vi "configuration UI.vi"() -> ()   [LabVIEW 2013, in "tag bus configurable plugin editor node.lvclass"]
uses:
  tag bus configurable plugin editor node.lvclass
  <vilib>/CEF_TreeControl/Node/NodeRef.ctl
  <vilib>/CEF_TreeControl/Node/NISE_CEF_Node.lvclass
  <vilib>/NI/AMC/Message Queue.ctl
  <vilib>/NI/AMC/Message.ctl
  <vilib>/NI/Tools/Keyed Array/KeyedArray.ctl
  <vilib>/CEF_TreeControl/Node/UserEventRef.ctl
  <vilib>/CEF_TreeControl/Controls/EventCluster.ctl
  module/configuration/tag bus configurable plugin module configuration.lvclass
  <vilib>/NI/Tag Bus Data Framework/Configuration Editor/Classes/Engine Parent/Engine Parent Editor Node.lvclass
  <vilib>/NI/Tag Bus/tag/tag descriptor.lvclass
  <vilib>/NI/Tag Bus/tag/Data Type.ctl
  <vilib>/NI/Module Execution Interface/Engine Configuration/engine configuration.lvclass
  <vilib>/NI/Tag Bus/tag/tag descriptor.lvclass/tag descriptor.ctl
  tag bus configurable plugin editor node.lvclass/tag bus configurable plugin editor node.ctl
  <vilib>/NI/Tag Bus Module Framework/root configuration/TBM configuration.lvclass/TBM configuration.ctl
  <vilib>/NI/Tag Bus/tag/write tag name.vi
  <vilib>/NI/Tag Bus/tag/write data type.vi
  <vilib>/NI/Tag Bus Module Framework/root configuration/create GUID.vi
  <vilib>/CEF_TreeControl/NISE_CEF_TreeControl.lvlib
  <vilib>/NI/Tag Bus Data Framework/Configuration Editor/Classes/Module editor node/module editor node.lvclass
  <vilib>/NI/Tag Bus Module Framework/channel/TBM channel.lvclass
  <vilib>/NI/Tag Bus Module Framework/root configuration/TBM configuration.lvclass
  <vilib>/NI/Tools/Keyed Array/Tools_KeyedArray.lvlib
  <vilib>/NI/AMC/AMC.lvlib
panel:
  in  "Tab Control":enum32{"Static Configuration"}(tab)
  in  "hidden_remove":bool
  in  "hidden_settings":bool
  in  "hidden_Add":bool
  in  "Remove Button":bool
  in  "Add Button":bool
  in  "channel":i32(listbox)
  in  "settings":bool
  in  "user event":T1
  in  "main queue":T2
  in  "node ref":T3
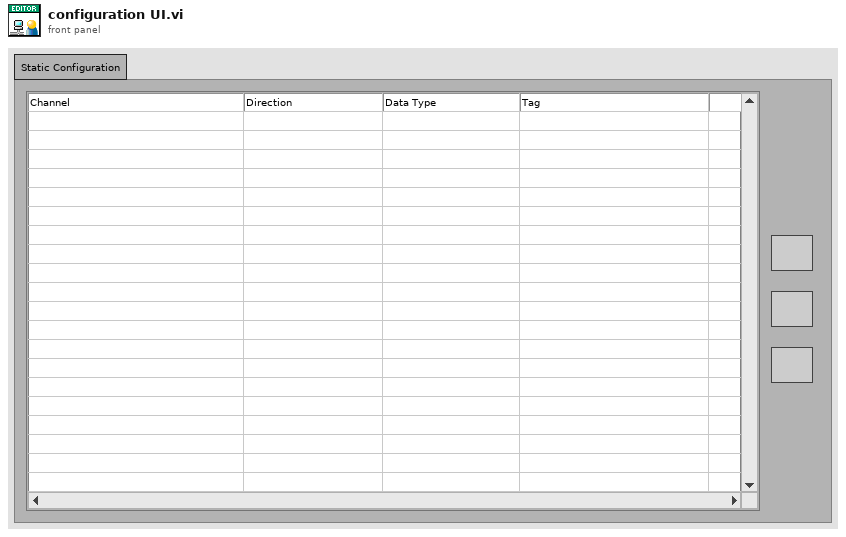
[diagram p1: front panel]
types:
  T1 = typedef "NISE_CEF_Node.lvclass/UserEventRef.ctl" = refnum<user-event>
  T2 = typedef "AMC.lvlib/Message Queue.ctl" = refnum<queue>
  T3 = typedef "NISE_CEF_Node.lvclass/NodeRef.ctl" = refnum<data-value>
  T4 = typedef "NISE_CEF_TreeControl.lvlib/EventCluster.ctl" = cluster{"command":string, "data":string}
  T5 = typedef "tag bus.lvlib/tag descriptor.lvclass/Data Type.ctl" = enum16{"Double", "Single", "I64", "I32", "I16", "I8", "U64", "U32", "U16", "U8", "Boolean", "String", "Array of Double", "Array of Single", "Array of I64", "Array of I32", "Array of I16", "Array of I8", "Array of U64", "Array of U32", "Array of U16", "Array of U8", "Array of Boolean", "Array of String"}
  T6 = typedef "tag bus configurable plugin editor node.lvclass/table line.ctl" = cluster{"channel":refnum<class "TBM channel.lvclass">, "tag name":string}
  T7 = typedef "LVPoint32TypeDef.ctl" = cluster{"Horizontal":i32, "Vertical":i32}
  T8 = typedef "LVRowAndColumnTypeDef.ctl" = cluster{"Row":i32, "Column":i32}
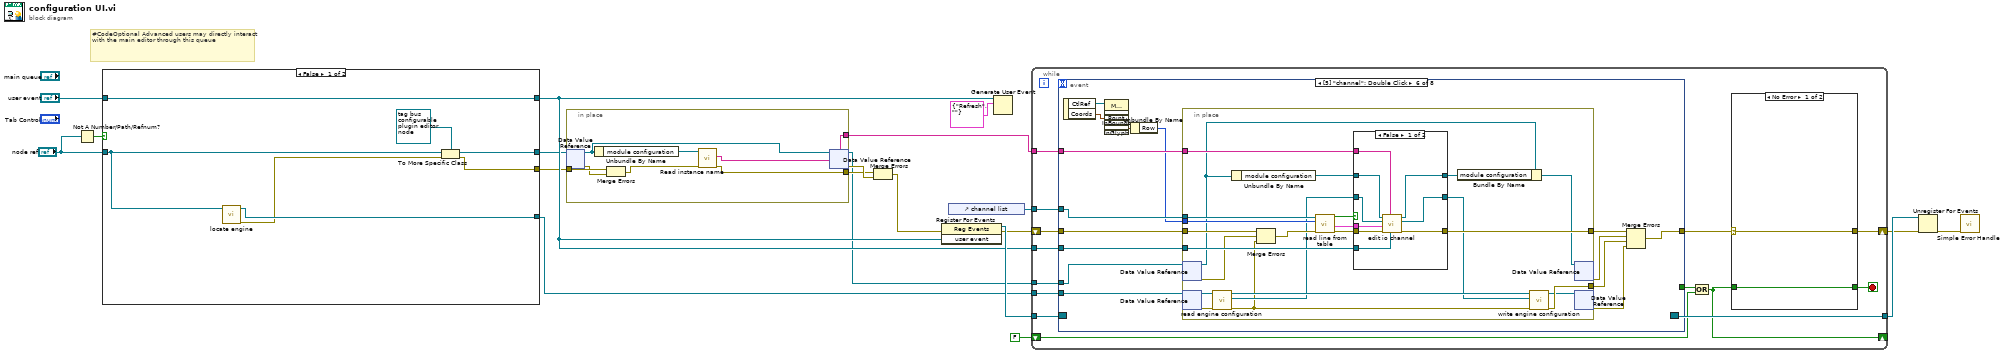
[diagram p0: block diagram]
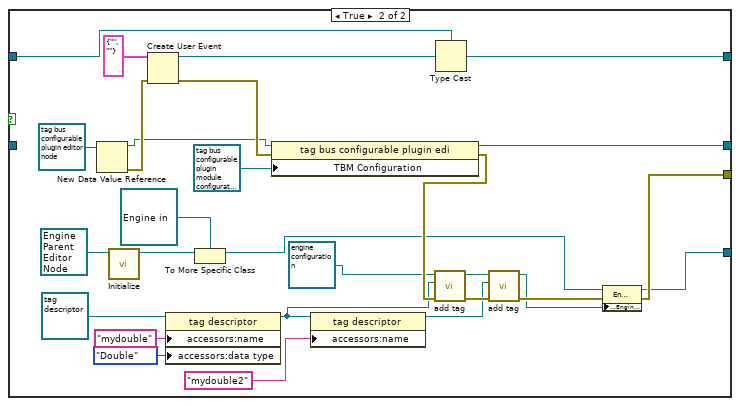
[diagram p2: hidden frame]
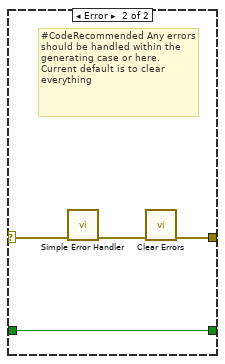
[diagram p3: hidden frame]
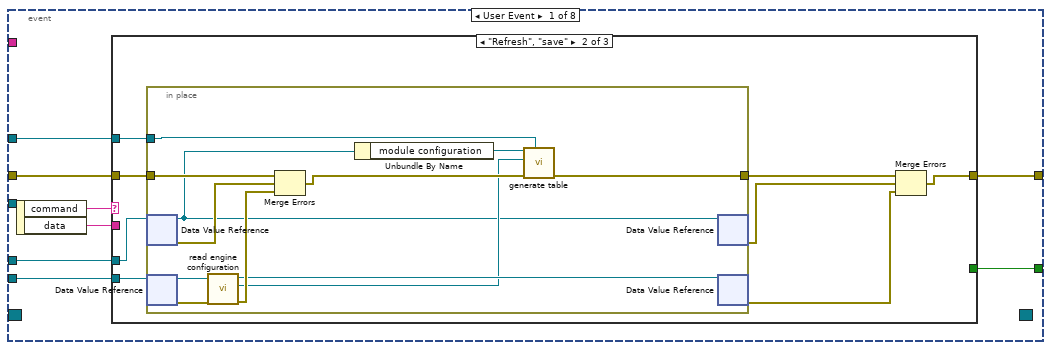
[diagram p4: hidden frame]
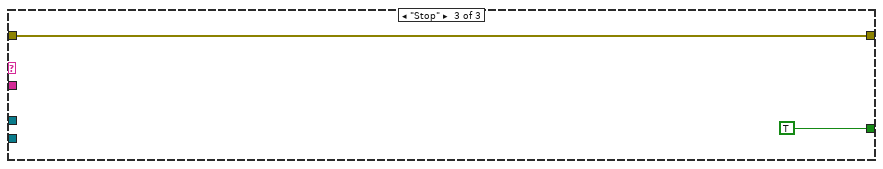
[diagram p6: hidden frame]
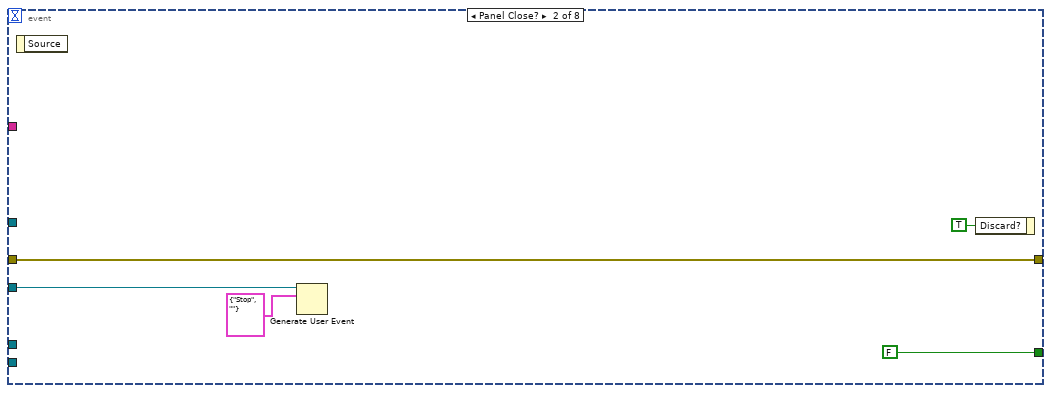
[diagram p7: hidden frame]
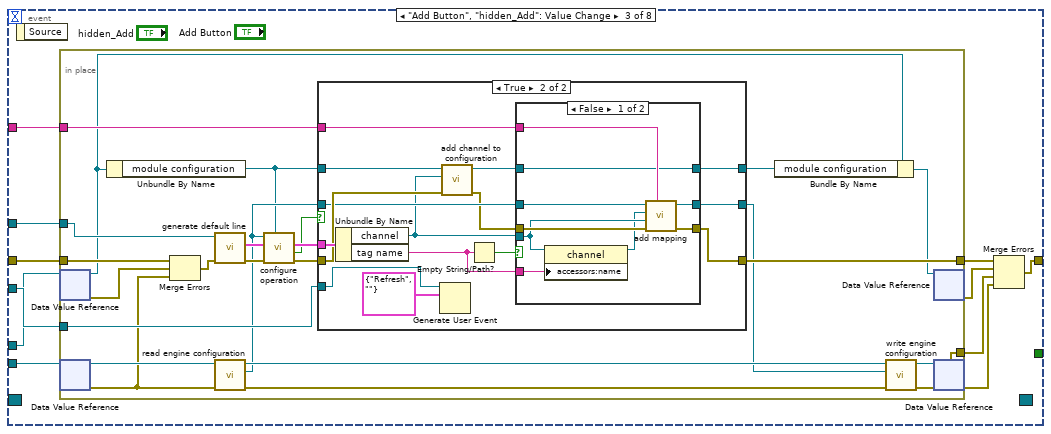
[diagram p8: hidden frame]
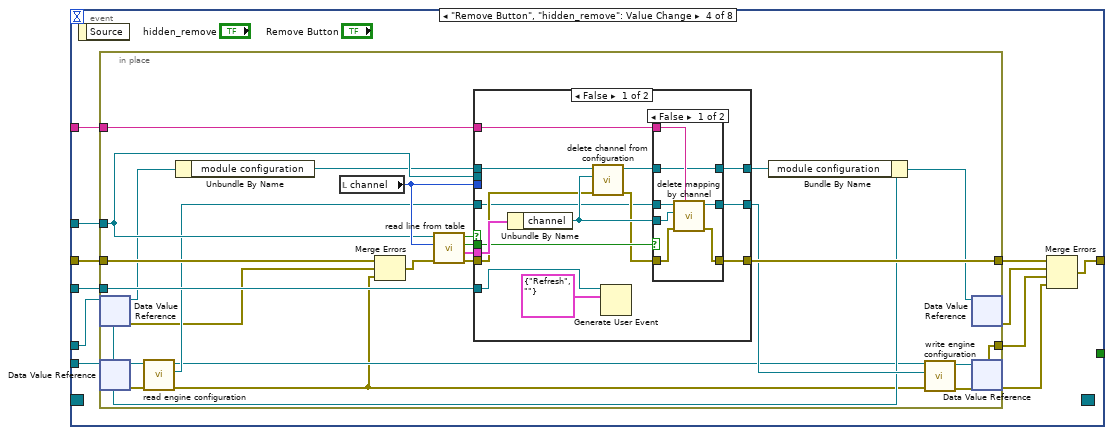
[diagram p11: hidden frame]
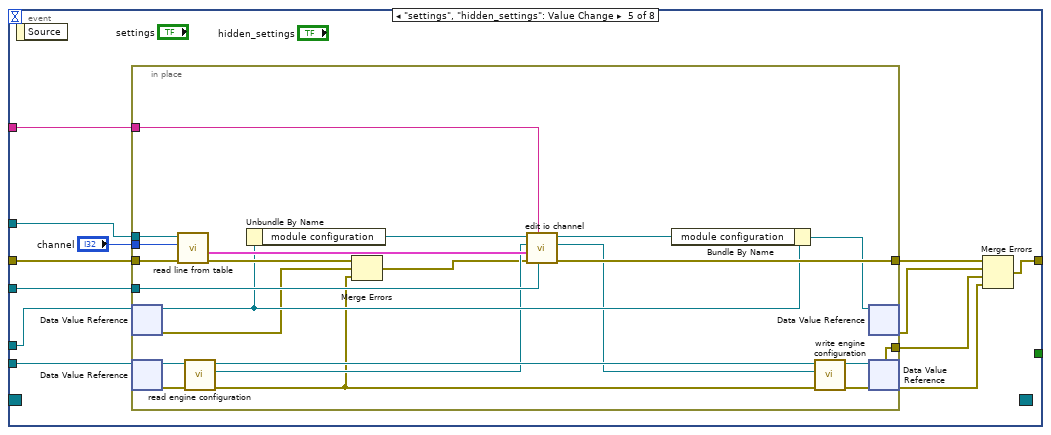
[diagram p14: hidden frame]
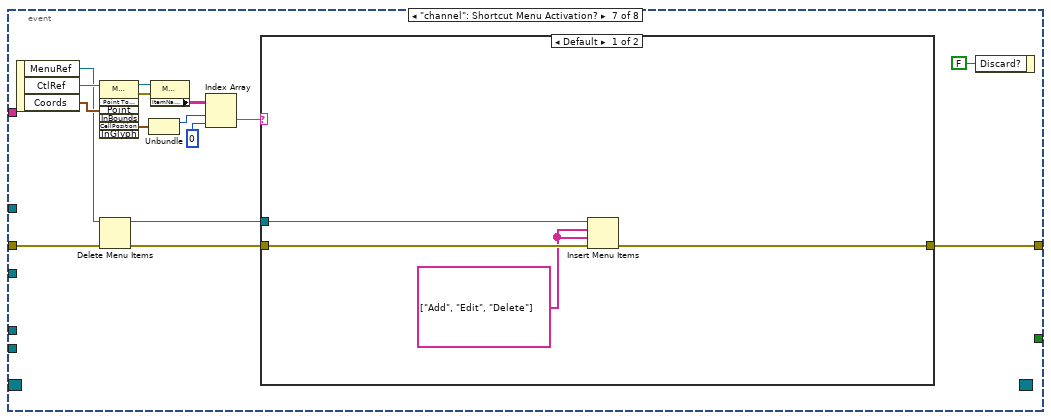
[diagram p16: hidden frame]
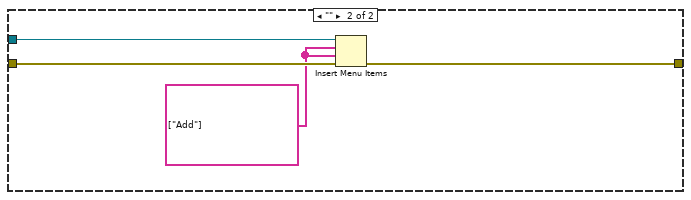
[diagram p17: hidden frame]
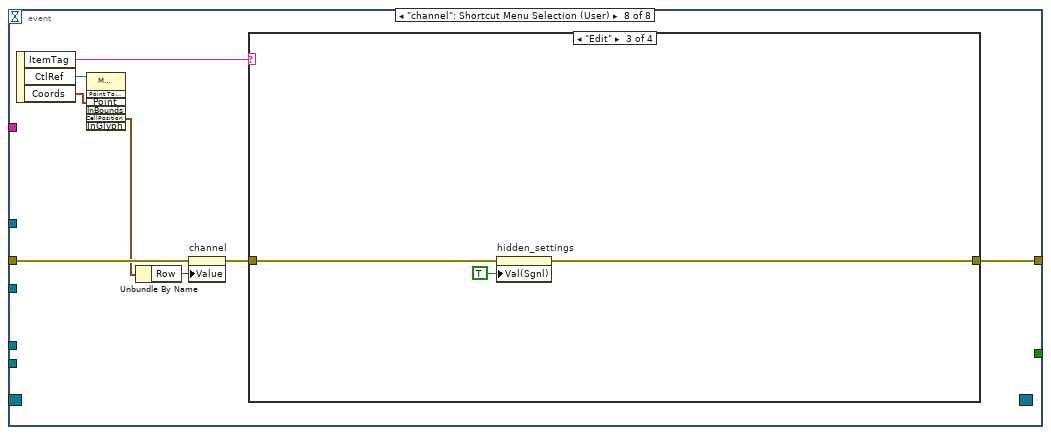
[diagram p18: hidden frame]
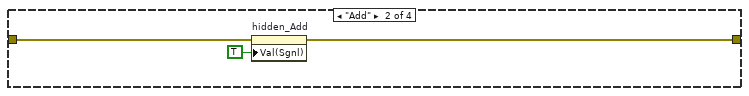
[diagram p20: hidden frame]
diagram:
  # "#CodeOptional Advanced users may directly interact with the main editor through this queue"
  n1 = Not A Number/Path/Refnum?(number/path/refnum="node ref") -> (NaN/Path/Refnum?=w16:bool)
  n2 = case shown="False" w16 {
    tunnel: "user event" -> [w27 w33]
    tunnel: [w27 w34] -> w8
    tunnel: "node ref" -> [w25 _]
    tunnel: [w24 w49] -> w7
    tunnel: [w23 w31] -> w6
    tunnel: [w22 w29] -> w12
    frame False {
      n3 = call <vilib>:"locate engine.vi"("component"=w25) -> ("error out"=w21:errorcluster, "engine"=w22:refnum<data-value>)  [unwired: 9 in]
      n4 = To More Specific Class(target class=refnum<data-value> refnum ("data value reference"), reference=w25, error in=w21) -> (specific class reference=w24:refnum<data-value>, error out=w23:errorcluster)
    }
    frame True {
      n5 = New Data Value Reference(data value=refnum<class "tag bus configurable plugin editor node.lvclass"> refnum ("tag bus configurable plugin editor node")) -> (data value reference=w48:refnum<data-value>, error out=w51:errorcluster)  [unwired: 1 in]
      n6 = call-dynamic "Initialize.vi"("Engine in"=refnum<class "Engine Parent Editor Node.lvclass"> refnum) -> ("data value reference"=w47:T3)  [unwired: 8 in, 2 out]
      n7 = Create User Event(user event datatype=T4 {"command"="", "data"=""} ("event data"), error in=w51) -> (user event=w54:refnum<user-event>, error out=w50:errorcluster)
      n8 = property class="tag descriptor"(reference=refnum<class "tag descriptor.lvclass"> refnum ("tag descriptor"), "accessors:name"="mydouble" ("name"), "accessors:data type"=Data_Type."Double" ("data type")) -> (reference out=w35:refnum<class "tag descriptor.lvclass">)  [unwired: 1 in, 1 out]
      n9 = To More Specific Class(target class=refnum<data-value> refnum ("data value reference"), reference=w47) -> (specific class reference=w30:refnum<data-value>)  [unwired: 1 in, 1 out]
      n10 = property class="tag bus configurable plugin edi"(reference=w48, error in=w50, "TBM Configuration"=refnum<class "tag bus configurable plugin module configuration.lvclass"> refnum ("tag bus configurable plugin module configuration")) -> (reference out=w49:refnum<data-value>, error out=w41:errorcluster)
      n11 = property class="tag descriptor"(reference=w35, "accessors:name"="mydouble2" ("name")) -> (reference out=w36:refnum<class "tag descriptor.lvclass">)  [unwired: 1 in, 1 out]
      n12 = call <vilib>:"add tag.vi"("error in"=w41, "tag descriptor"=w35, "engine configuration in"=refnum<class "engine configuration.lvclass"> refnum ("Engine Configuration")) -> ("error out"=w39:errorcluster, "engine configuration out"=w38:refnum<class "engine configuration.lvclass">)  [unwired: 7 in]
      n13 = Type Cast(type=w33, x=w54) -> (*(type *) &x=w34:T1)
      n14 = call <vilib>:"add tag.vi"("error in"=w39, "tag descriptor"=w36, "engine configuration in"=w38) -> ("error out"=w37:errorcluster, "engine configuration out"=w28:refnum<class "engine configuration.lvclass">)  [unwired: 7 in]
      n15 = property class="Engine Parent Editor Node.lvcla"(reference=w30, error in=w37, "Data Access:Engine Configuration"=w28) -> (reference out=w29:refnum<data-value>, error out=w31:errorcluster)
    }
  }
  n16 = in-place {
    in-place-border: w6 -> [w62]
    in-place-border: [w57] -> w4
    in-place-border: [w56] -> w2
    n17 = in-place-dvr #1(w7) -> (w60:refnum<class "tag bus configurable plugin editor node.lvclass">, w61:errorcluster)
    n18 = Unbundle By Name(w60) -> ("module configuration"=w59:refnum<class "tag bus configurable plugin module configuration.lvclass">)
    n19 = Merge Errors(w62, w61) -> (w58:errorcluster)
    n20 = call <vilib>:"Read instance name.vi"("error in"=w58, "configuration in"=w59) -> ("error out"=w57:errorcluster, "instance id"=w56:string)  [unwired: 7 in, 1 out]
    n21 = in-place-dvr #1(w60) -> (w1:refnum<data-value>, w5:errorcluster)
  }
  n22 = Merge Errors(w4, w5) -> (w3:errorcluster)
  n23 = register-events(error in=w3, w8) -> (reference out=w20:refnum<event-registration>, error out=w13:errorcluster)  [unwired: 1 in]
  n24 = control-ref of="channel list"() -> (w10:refnum<vi>)
  n25 = Generate User Event(user event=w8, event data cluster=T4 {"command"="Refresh", "data"=""} ("event data")) -> ()  [unwired: 2 in, 2 out]
  n26 = while {
    tunnel: w20 -> [w76]
    tunnel: [w75] -> w19
    shift-right: [w69] -> w18
    shift-left: w13 -> [w74]
    shift-right: [w71] -> _
    shift-left: FALSE -> [w70]
    tunnel: w2 -> [w68]
    tunnel: w1 -> [w67]
    tunnel: w12 -> [w66]
    tunnel: w8 -> [w65]
    tunnel: w10 -> [w63]
    stop <- w73 stop-if-true
    n27 = event shown="[5] \"channel\": Double Click" {
      selector: w76 -> [_ _ _ _ _ _ _ _]
      dyn-events: [_ _ _ _ _ _ _ _] -> w75
      timeout: _ -> [_ _ _ _ _ _ _ _]
      tunnel: [w90 FALSE _ _ _ _ _ _] -> w72
      tunnel: [w84 w117 w124 w188 w251 w285 w330 w357] -> w64
      tunnel: w74 -> [w85 w117 w128 w193 w257 w294 w344 w356]
      tunnel: w68 -> [_ _ w127 w192 w254 w292 _ _]
      tunnel: w67 -> [w88 _ w122 w184 w249 w281 _ _]
      tunnel: w66 -> [w87 _ w123 w189 w250 w282 _ _]
      tunnel: w65 -> [_ w114 w126 w191 w253 w291 _ _]
      tunnel: w63 -> [w83 _ w125 w190 w252 w290 _ _]
      event User Event {
        n28 = event-data() -> ("command"=w89:string, "data"=w86:string)  [unwired: 1 in]
        n29 = case shown="\"Refresh\", \"save\"" w89 {
          tunnel: [_ _ TRUE] -> w90
          tunnel: w88 -> [_ w95 _]
          tunnel: w87 -> [_ w96 _]
          tunnel: w86 -> [_ _ _]
          tunnel: w85 -> [w91 w99 w112]
          tunnel: [w91 w94 w112] -> w84
          tunnel: w83 -> [_ w97 _]
          frame Default {
          }
          frame "Refresh", "save" {
            n30 = in-place {
              in-place-border: w99 -> [w111]
              in-place-border: [w110] -> w98
              in-place-border: w97 -> [w109]
              n31 = in-place-dvr #2(w95) -> (w101:refnum<class "tag bus configurable plugin editor node.lvclass">, w107:errorcluster)
              n32 = in-place-dvr #3(w96) -> (w104:refnum<class "Engine Parent Editor Node.lvclass">, w106:errorcluster)
              n33 = call <vilib>:"read engine configuration.vi"("error in"=w106, "Engine Parent Editor Node in"=w104) -> ("error out"=w105:errorcluster, "engine configuration"=w102:refnum<class "engine configuration.lvclass">, "Engine Parent Editor Node out"=w103:refnum<class "Engine Parent Editor Node.lvclass">)  [unwired: 7 in]
              n34 = Merge Errors(w111, w107, w105) -> (w108:errorcluster)
              n35 = Unbundle By Name(w101) -> ("module configuration"=w100:refnum<class "tag bus configurable plugin module configuration.lvclass">)
              n36 = call "generate table.vi"("table"=w109, "error in"=w108, "engine configuration"=w102, "tag bus configurable plugin module configuration"=w100) -> ("error out"=w110:errorcluster)  [unwired: 7 in]
              n37 = in-place-dvr #2(w101) -> (w93:errorcluster)  [unwired: 1 out]
              n38 = in-place-dvr #3(w103) -> (w92:errorcluster)  [unwired: 1 out]
            }
            n39 = Merge Errors(w98, w93, w92) -> (w94:errorcluster)
          }
          frame "Stop" {
          }
        }
      }
      event Panel Close? {
        n40 = event-data() -> ()  [unwired: 1 in, 1 out]
        n41 = Generate User Event(user event=w114, event data cluster=T4 {"command"="Stop", "data"=""} ("event data")) -> ()  [unwired: 2 in, 2 out]
        n42 = event-data("Discard?"=TRUE) -> ()  [unwired: 1 in, 1 out]
      }
      event "Add Button", "hidden_Add": Value Change {
        n43 = event-data() -> ()  [unwired: 1 in, 1 out]
        n44 = in-place {
          in-place-border: [w153] -> w129
          in-place-border: w128 -> [w152]
          in-place-border: w127 -> [w147]
          in-place-border: w126 -> [w145]
          in-place-border: w125 -> [w144]
          in-place-border: [w139] -> w120
          n45 = in-place-dvr #4(w122) -> (w132:refnum<class "tag bus configurable plugin editor node.lvclass">, w133:errorcluster)
          n46 = in-place-dvr #5(w123) -> (w142:refnum<class "Engine Parent Editor Node.lvclass">, w141:errorcluster)
          n47 = Unbundle By Name(w132) -> ("module configuration"=w134:refnum<class "tag bus configurable plugin module configuration.lvclass">)
          n48 = Merge Errors(w152, w133, w141) -> (w143:errorcluster)
          n49 = call "generate default line.vi"("error in"=w143, "operations table"=w144) -> ("error out"=w150:errorcluster, "line"=w151:T6)  [unwired: 8 in]
          n50 = call <vilib>:"read engine configuration.vi"("error in"=w141, "Engine Parent Editor Node in"=w142) -> ("error out"=w137:errorcluster, "engine configuration"=w135:refnum<class "engine configuration.lvclass">, "Engine Parent Editor Node out"=w138:refnum<class "Engine Parent Editor Node.lvclass">)  [unwired: 7 in]
          n51 = call "configure operation.vi"("tag bus configurable plugin module configuration"=w134, "error in"=w150, "line item in"=w151, "engine configuration"=w135) -> ("error out"=w148:errorcluster, "success"=w146:bool, "line item out"=w149:T6)  [unwired: 4 in, 1 out]
          n52 = case shown="True" w146 {
            tunnel: [w156 w159] -> w153
            tunnel: w148 -> [w156 w169]
            tunnel: w135 -> [w155 w167]
            tunnel: w149 -> [_ w170]
            tunnel: w134 -> [w154 w171]
            tunnel: [w155 w166] -> w136
            tunnel: [w154 w160] -> w131
            tunnel: w147 -> [_ w163]
            tunnel: w145 -> [_ w158]
            frame False {
            }
            frame True {
              n53 = Unbundle By Name(w170) -> ("channel"=w164:refnum<class "TBM channel.lvclass">, "tag name"=w162:string)
              n54 = Generate User Event(user event=w158, event data cluster=T4 {"command"="Refresh", "data"=""} ("event data")) -> ()  [unwired: 2 in, 2 out]
              n55 = call "add channel to configuration.vi"("error in"=w169, "channel"=w164, "tag bus configurable plugin module configuration in"=w171) -> ("error out"=w165:errorcluster, "tag bus configurable plugin module configuration out"=w161:refnum<class "tag bus configurable plugin module configuration.lvclass">)  [unwired: 7 in]
              n56 = Empty String/Path?(string/path=w162) -> (empty?=w168:bool)
              n57 = case shown="False" w168 {
                tunnel: w167 -> [w180 w183]
                tunnel: [w179 w183] -> w166
                tunnel: w165 -> [w178 w182]
                tunnel: w164 -> [w176 _]
                tunnel: w163 -> [w177 _]
                tunnel: w162 -> [w175 _]
                tunnel: [w173 w182] -> w159
                tunnel: w161 -> [w172 w181]
                tunnel: [w172 w181] -> w160
                frame False {
                  n58 = property class="channel"(reference=w176, "accessors:name"=w175) -> (reference out=w174:refnum<class "TBM channel.lvclass">)  [unwired: 1 in, 1 out]
                  n59 = call <vilib>:"add mapping.vi"("owner ID"=w177, "error in"=w178, "channel"=w176, "tag descriptor"=w174, "engine configuration"=w180) -> ("error out"=w173:errorcluster, "engine configuration out"=w179:refnum<class "engine configuration.lvclass">)  [unwired: 5 in]
                }
                frame True {
                }
              }
            }
          }
          n60 = Bundle By Name(cluster=w132, "module configuration"=w131) -> (w130:refnum<class "tag bus configurable plugin editor node.lvclass">)
          n61 = call <vilib>:"write engine configuration.vi"("error in"=w137, "engine configuration"=w136, "Engine Parent Editor Node in"=w138) -> ("error out"=w139:errorcluster, "Engine Parent Editor Node out"=w140:refnum<class "Engine Parent Editor Node.lvclass">)  [unwired: 7 in]
          n62 = in-place-dvr #4(w130) -> (w119:errorcluster)  [unwired: 1 out]
          n63 = in-place-dvr #5(w140) -> (w121:errorcluster)  [unwired: 1 out]
        }
        n64 = Merge Errors(w129, w119, w120, w121) -> (w124:errorcluster)
      }
      event "Remove Button", "hidden_remove": Value Change {
        n65 = event-data() -> ()  [unwired: 1 in, 1 out]
        n66 = in-place {
          in-place-border: [w218] -> w194
          in-place-border: w193 -> [w217]
          in-place-border: w192 -> [w211]
          in-place-border: w191 -> [w210]
          in-place-border: w190 -> [w209]
          in-place-border: [w207] -> w185
          n67 = in-place-dvr #6(w184) -> (w200:refnum<class "tag bus configurable plugin editor node.lvclass">, w195:errorcluster)
          n68 = in-place-dvr #7(w189) -> (w203:refnum<class "Engine Parent Editor Node.lvclass">, w202:errorcluster)
          n69 = call <vilib>:"read engine configuration.vi"("error in"=w202, "Engine Parent Editor Node in"=w203) -> ("error out"=w196:errorcluster, "engine configuration"=w198:refnum<class "engine configuration.lvclass">, "Engine Parent Editor Node out"=w197:refnum<class "Engine Parent Editor Node.lvclass">)  [unwired: 7 in]
          n70 = Unbundle By Name(w200) -> ("module configuration"=w199:refnum<class "tag bus configurable plugin module configuration.lvclass">)
          n71 = local read "channel"() -> (w216:i32)
          n72 = Merge Errors(w217, w195, w196) -> (w201:errorcluster)
          n73 = call "read line from table.vi"("error in"=w201, "line number"=w216, "channels table"=w209) -> ("error out"=w212:errorcluster, "line"=w215:T6, "empty tag?"=w213:bool, "empty channel?"=w214:bool)  [unwired: 5 in]
          n74 = case shown="False" w214 {
            tunnel: [w221 w244] -> w218
            tunnel: w216 -> [_ _]
            tunnel: w209 -> [_ _]
            tunnel: w215 -> [w232 _]
            tunnel: w199 -> [w230 w243]
            tunnel: w198 -> [w225 w245]
            tunnel: w213 -> [w231 _]
            tunnel: w212 -> [w228 w244]
            tunnel: w211 -> [w224 _]
            tunnel: [w223 w245] -> w204
            tunnel: [w222 w243] -> w205
            tunnel: w210 -> [w219 _]
            frame False {
              n75 = Unbundle By Name(w232) -> ("channel"=w229:refnum<class "TBM channel.lvclass">)
              n76 = call "delete channel from configuration.vi"("error in"=w228, "channel"=w229, "tag bus configurable plugin module configuration in"=w230) -> ("error out"=w226:errorcluster, "tag bus configurable plugin module configuration out"=w227:refnum<class "tag bus configurable plugin module configuration.lvclass">)  [unwired: 7 in]
              n77 = Generate User Event(user event=w219, event data cluster=T4 {"command"="Refresh", "data"=""} ("event data")) -> ()  [unwired: 2 in, 2 out]
              n78 = case shown="False" w231 {
                tunnel: w229 -> [w238 _]
                tunnel: w227 -> [w233 w240]
                tunnel: w226 -> [w236 w241]
                tunnel: w225 -> [w239 w242]
                tunnel: w224 -> [w237 _]
                tunnel: [w235 w242] -> w223
                tunnel: [w234 w241] -> w221
                tunnel: [w233 w240] -> w222
                frame False {
                  n79 = call <vilib>:"delete mapping by channel.vi"("owner ID"=w237, "error in"=w236, "channel"=w238, "engine configuration in"=w239) -> ("error out"=w234:errorcluster, "engine configuration out"=w235:refnum<class "engine configuration.lvclass">)  [unwired: 6 in]
                }
                frame True {
                }
              }
            }
            frame True {
            }
          }
          n80 = Bundle By Name(cluster=w200, "module configuration"=w205) -> (w206:refnum<class "tag bus configurable plugin editor node.lvclass">)
          n81 = call <vilib>:"write engine configuration.vi"("error in"=w196, "engine configuration"=w204, "Engine Parent Editor Node in"=w197) -> ("error out"=w207:errorcluster, "Engine Parent Editor Node out"=w208:refnum<class "Engine Parent Editor Node.lvclass">)  [unwired: 7 in]
          n82 = in-place-dvr #6(w206) -> (w186:errorcluster)  [unwired: 1 out]
          n83 = in-place-dvr #7(w208) -> (w187:errorcluster)  [unwired: 1 out]
        }
        n84 = Merge Errors(w194, w186, w185, w187) -> (w188:errorcluster)
      }
      event "settings", "hidden_settings": Value Change {
        n85 = event-data() -> ()  [unwired: 1 in, 1 out]
        n86 = in-place {
          in-place-border: w257 -> [w279]
          in-place-border: [w278] -> w256
          in-place-border: "channel" -> [w275]
          in-place-border: w254 -> [w274]
          in-place-border: w253 -> [w273]
          in-place-border: w252 -> [w272]
          in-place-border: [w265] -> w246
          n87 = in-place-dvr #8(w249) -> (w271:refnum<class "tag bus configurable plugin editor node.lvclass">, w258:errorcluster)
          n88 = in-place-dvr #9(w250) -> (w268:refnum<class "Engine Parent Editor Node.lvclass">, w267:errorcluster)
          n89 = call "read line from table.vi"("error in"=w279, "line number"=w275, "channels table"=w272) -> ("error out"=w277:errorcluster, "line"=w276:T6)  [unwired: 5 in, 2 out]
          n90 = call <vilib>:"read engine configuration.vi"("error in"=w267, "Engine Parent Editor Node in"=w268) -> ("error out"=w259:errorcluster, "engine configuration"=w261:refnum<class "engine configuration.lvclass">, "Engine Parent Editor Node out"=w263:refnum<class "Engine Parent Editor Node.lvclass">)  [unwired: 7 in]
          n91 = Unbundle By Name(w271) -> ("module configuration"=w264:refnum<class "tag bus configurable plugin module configuration.lvclass">)
          n92 = Merge Errors(w277, w258, w259) -> (w260:errorcluster)
          n93 = call "edit io channel.vi"("user event"=w273, "Properties:instance identifier"=w274, "error in"=w260, "line"=w276, "engine configuration in"=w261, "tag bus configurable plugin module configuration in"=w264) -> ("error out"=w278:errorcluster, "engine configuration"=w262:refnum<class "engine configuration.lvclass">, "tag bus configurable plugin module configuration out"=w269:refnum<class "tag bus configurable plugin module configuration.lvclass">)  [unwired: 3 in]
          n94 = Bundle By Name(cluster=w271, "module configuration"=w269) -> (w270:refnum<class "tag bus configurable plugin editor node.lvclass">)
          n95 = call <vilib>:"write engine configuration.vi"("error in"=w259, "engine configuration"=w262, "Engine Parent Editor Node in"=w263) -> ("error out"=w265:errorcluster, "Engine Parent Editor Node out"=w266:refnum<class "Engine Parent Editor Node.lvclass">)  [unwired: 7 in]
          n96 = in-place-dvr #8(w270) -> (w247:errorcluster)  [unwired: 1 out]
          n97 = in-place-dvr #9(w266) -> (w248:errorcluster)  [unwired: 1 out]
        }
        n98 = Merge Errors(w256, w247, w246, w248) -> (w251:errorcluster)
      }
      event "channel": Double Click {
        n99 = event-data() -> ("CtlRef"=w289:refnum<vi>, "Coords"=w288:T7)  [unwired: 1 in]
        n100 = invoke class="MCListbox (strict)" method="Point To Row Column"(reference=w289, "Point"=w288) -> ("CellPosition"=w287:T8)  [unwired: 5 in, 6 out]
        n101 = Unbundle By Name(w287) -> ("Row"=w286:i32)
        n102 = in-place {
          in-place-border: w294 -> [w317]
          in-place-border: [w316] -> w293
          in-place-border: w292 -> [w313]
          in-place-border: w291 -> [w312]
          in-place-border: w290 -> [w311]
          in-place-border: w286 -> [w310]
          in-place-border: [w307] -> w280
          n103 = in-place-dvr #10(w281) -> (w296:refnum<class "tag bus configurable plugin editor node.lvclass">, w301:errorcluster)
          n104 = in-place-dvr #11(w282) -> (w305:refnum<class "Engine Parent Editor Node.lvclass">, w304:errorcluster)
          n105 = call <vilib>:"read engine configuration.vi"("error in"=w304, "Engine Parent Editor Node in"=w305) -> ("error out"=w300:errorcluster, "engine configuration"=w302:refnum<class "engine configuration.lvclass">, "Engine Parent Editor Node out"=w303:refnum<class "Engine Parent Editor Node.lvclass">)  [unwired: 7 in]
          n106 = Unbundle By Name(w296) -> ("module configuration"=w295:refnum<class "tag bus configurable plugin module configuration.lvclass">)
          n107 = Merge Errors(w317, w301, w300) -> (w308:errorcluster)
          n108 = call "read line from table.vi"("error in"=w308, "line number"=w310, "channels table"=w311) -> ("error out"=w315:errorcluster, "line"=w314:T6, "empty channel?"=w309:bool)  [unwired: 5 in, 1 out]
          n109 = case shown="False" w309 {
            tunnel: [w326 w327] -> w316
            tunnel: w315 -> [w325 w327]
            tunnel: w314 -> [w324 _]
            tunnel: w302 -> [w323 w328]
            tunnel: w295 -> [w322 w329]
            tunnel: [w321 w329] -> w298
            tunnel: [w320 w328] -> w299
            tunnel: w313 -> [w319 _]
            tunnel: w312 -> [w318 _]
            frame False {
              n110 = call "edit io channel.vi"("user event"=w318, "Properties:instance identifier"=w319, "error in"=w325, "line"=w324, "engine configuration in"=w323, "tag bus configurable plugin module configuration in"=w322) -> ("error out"=w326:errorcluster, "engine configuration"=w320:refnum<class "engine configuration.lvclass">, "tag bus configurable plugin module configuration out"=w321:refnum<class "tag bus configurable plugin module configuration.lvclass">)  [unwired: 3 in]
            }
            frame True {
            }
          }
          n111 = Bundle By Name(cluster=w296, "module configuration"=w298) -> (w297:refnum<class "tag bus configurable plugin editor node.lvclass">)
          n112 = call <vilib>:"write engine configuration.vi"("error in"=w300, "engine configuration"=w299, "Engine Parent Editor Node in"=w303) -> ("error out"=w307:errorcluster, "Engine Parent Editor Node out"=w306:refnum<class "Engine Parent Editor Node.lvclass">)  [unwired: 7 in]
          n113 = in-place-dvr #10(w297) -> (w283:errorcluster)  [unwired: 1 out]
          n114 = in-place-dvr #11(w306) -> (w284:errorcluster)  [unwired: 1 out]
        }
        n115 = Merge Errors(w293, w283, w280, w284) -> (w285:errorcluster)
      }
      event "channel": Shortcut Menu Activation? {
        n116 = event-data() -> ("MenuRef"=w340:refnum<k9>, "CtlRef"=w342:refnum<vi>, "Coords"=w341:T7)  [unwired: 1 in]
        n117 = invoke class="MCListbox (strict)" method="Point To Row Column"(reference=w342, "Point"=w341) -> (reference out=w339:refnum<vi>, error out=w338:errorcluster, "CellPosition"=w337:T8)  [unwired: 5 in, 4 out]
        n118 = Delete Menu Items(6:w344, 9:w340) -> (0:w331:errorcluster, 3:w332:refnum<k9>)  [unwired: 2 in]
        n119 = Unbundle(w337) -> ("Row"=w335:i32)  [unwired: 1 out]
        n120 = property class="MCListbox (strict)"(reference=w339, error in=w338) -> ("ItemNames"=w336:string[][])  [unwired: 2 out]
        n121 = Index Array(array=w336, index (row)=w335, index (col)=0 ("disabled index (col)")) -> (element=w333:string)
        n122 = case shown="Default" w333 {
          tunnel: w332 -> [w348 w352]
          tunnel: w331 -> [w347 w351]
          tunnel: [w346 w350] -> w330
          frame Default {
            w345 = string[] ["Add", "Edit", "Delete"] ("item names")
            n123 = Insert Menu Items(6:w347, 7:w345, 8:w345, 9:w348) -> (0:w346:errorcluster)  [unwired: 2 in, 2 out]
          }
          frame "" {
            w349 = string[] ["Add"] ("item names")
            n124 = Insert Menu Items(6:w351, 7:w349, 8:w349, 9:w352) -> (0:w350:errorcluster)  [unwired: 2 in, 2 out]
          }
        }
        n125 = event-data("Discard?"=FALSE) -> ()  [unwired: 1 in, 1 out]
      }
      event "channel": Shortcut Menu Selection (User) {
        n126 = event-data() -> ("ItemTag"=w358:string, "CtlRef"=w359:refnum<vi>, "Coords"=w360:T7)  [unwired: 1 in]
        n127 = invoke class="MCListbox (strict)" method="Point To Row Column"(reference=w359, "Point"=w360) -> ("CellPosition"=w354:T8)  [unwired: 5 in, 6 out]
        n128 = Unbundle By Name(w354) -> ("Row"=w353:i32)
        n129 = property on="channel" class="MCListbox (strict)"(error in=w356, "Value"=w353) -> (error out=w355:errorcluster)  [unwired: 1 in, 1 out]
        n130 = case shown="\"Edit\"" w358 {
          tunnel: w355 -> [w361 w363 w367 w370]
          tunnel: [w361 w362 w366 w369] -> w357
          frame Default {
          }
          frame "Add" {
            n131 = property on="hidden_Add" class="Bool (strict)"(error in=w363, "Val(Sgnl)"=TRUE ("Value (Signaling)")) -> (error out=w362:errorcluster)  [unwired: 1 in, 1 out]
          }
          frame "Edit" {
            n132 = property on="hidden_settings" class="Bool (strict)"(error in=w367, "Val(Sgnl)"=TRUE ("Value (Signaling)")) -> (error out=w366:errorcluster)  [unwired: 1 in, 1 out]
          }
          frame "Delete" {
            n133 = property on="hidden_remove" class="Bool (strict)"(error in=w370, "Val(Sgnl)"=FALSE ("Value (Signaling)")) -> (error out=w369:errorcluster)  [unwired: 1 in, 1 out]
          }
        }
      }
    }
    n134 = Or(x=w72, y=w70) -> (x .or. y?=w71:bool)
    n135 = case shown="No Error" w64 {
      selector: w64 -> [w77 w81]
      tunnel: [w78 w82] -> w73
      tunnel: w71 -> [w78 w82]
      tunnel: [w77 w79] -> w69
      frame No Error {
      }
      frame Error {
        # "#CodeRecommended Any errors should be handled within the generating case or here. Current default is to clear everything"
        n136 = call <vilib>:"Simple Error Handler.vi"("error in (no error)"=w81) -> ("error out"=w80:errorcluster)  [unwired: 4 in, 4 out]
        n137 = call <vilib>:"Clear Errors.vi"("error in (no error)"=w80) -> ("error out"=w79:errorcluster)  [unwired: 6 in]
      }
    }
  }
  n138 = Unregister For Events(event registration refnum=w19, error in=w18) -> (error out=w11:errorcluster)
  n139 = call <vilib>:"Simple Error Handler.vi"("error in (no error)"=w11) -> ()  [unwired: 4 in, 5 out]
